vi "per socket initialization.vi"(7 "id":i32, 8 "error in":errorcluster, 10 "upgrade data":T1, 11 "websocket user plugin in":refnum<class "websocket user plugin.lvclass">) -> (0 "error out":errorcluster, 3 "websocket user plugin out":refnum<class "websocket user plugin.lvclass">)   [LabVIEW 2016, in "websocket user plugin.lvclass"]
uses:
  websocket user plugin.lvclass
  HTTP responder/http upgrade data.ctl
  HTTP server/http request.ctl
  HTTP server/http method.ctl
  HTTP headers/http header data.ctl
  HTTP server/Basic HTTP server.lvclass
  HTTP responder/http responder.lvclass
  HTTP headers/http headers.lvlib
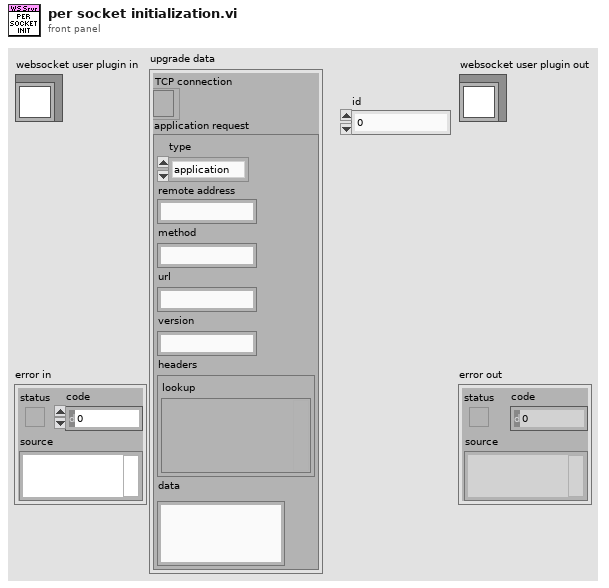
[diagram p1: front panel]
types:
  T1 = typedef "http responder.lvclass/http upgrade data.ctl" = cluster{"TCP connection":refnum<k5>, "application request":T2}
  T2 = typedef "Basic HTTP server.lvclass/http request.ctl" = cluster{"type":T3, "remote address":string, "method":string, "url":string, "version":string, "headers":T4, "data":string}
  T3 = typedef "Basic HTTP server.lvclass/http method.ctl" = enum16{"application", "error", "upgrade", "expect"}
  T4 = typedef "http headers.lvlib/http header data.ctl" = cluster{"lookup":variant}
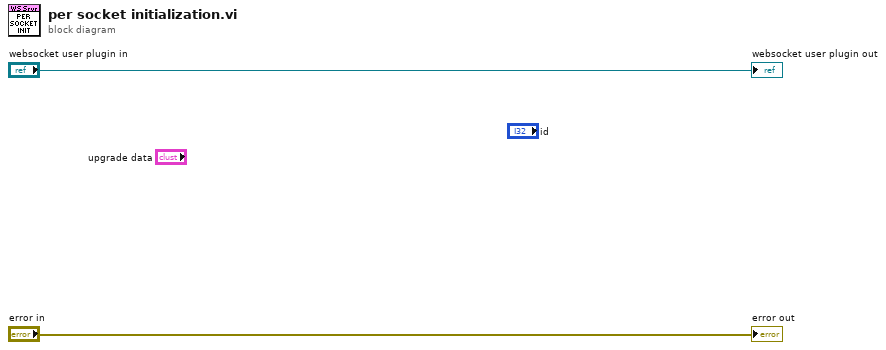
[diagram p0: block diagram]
diagram:
  "error out" <- "error in"
  "websocket user plugin out" <- "websocket user plugin in"
